vi "SEWV Specific Enthalpy of Water Vapor Revised (J to Kg).vi"(2 "Partial Pressure of Water Vapor":dbl[unit], 3 "Tceg":dbl[unit]) -> (0 "Spesific Valume":dbl[unit], 1 "SEWV":dbl[unit])   [LabVIEW 2018]
panel:
  out "Spesific Vaolume":dbl[unit](slide) scale=0.0..100.0
  out "SEWV":dbl[unit](knob) scale=0.0..6000000.0
  out "DriveGamaRTconstant":dbl
  out "DriveGama0Tconstant":dbl
  out "DriveGamaRPconstant":dbl
  out "Partial Presure of Water Vapor":dbl[unit](knob) scale=0.0..2.0
  out "Temprature of Humid Air\nKelvin Degree":dbl[unit](slide) scale=273.0..373.0
  out "Tk":dbl[unit]
  out "DriveGama0Pconstant":dbl
  out "Temprature of Humid Air\nCentigrade Degree":dbl[unit](slide) scale=0.0..100.0
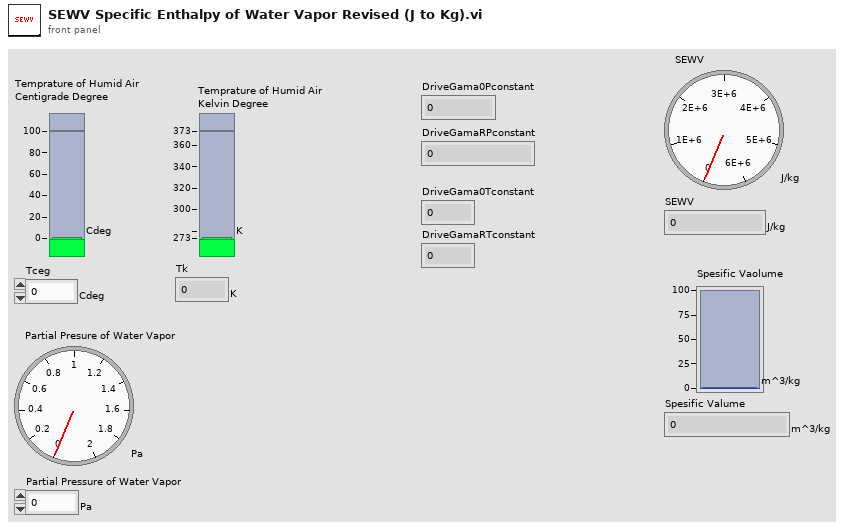
[diagram p1: front panel]
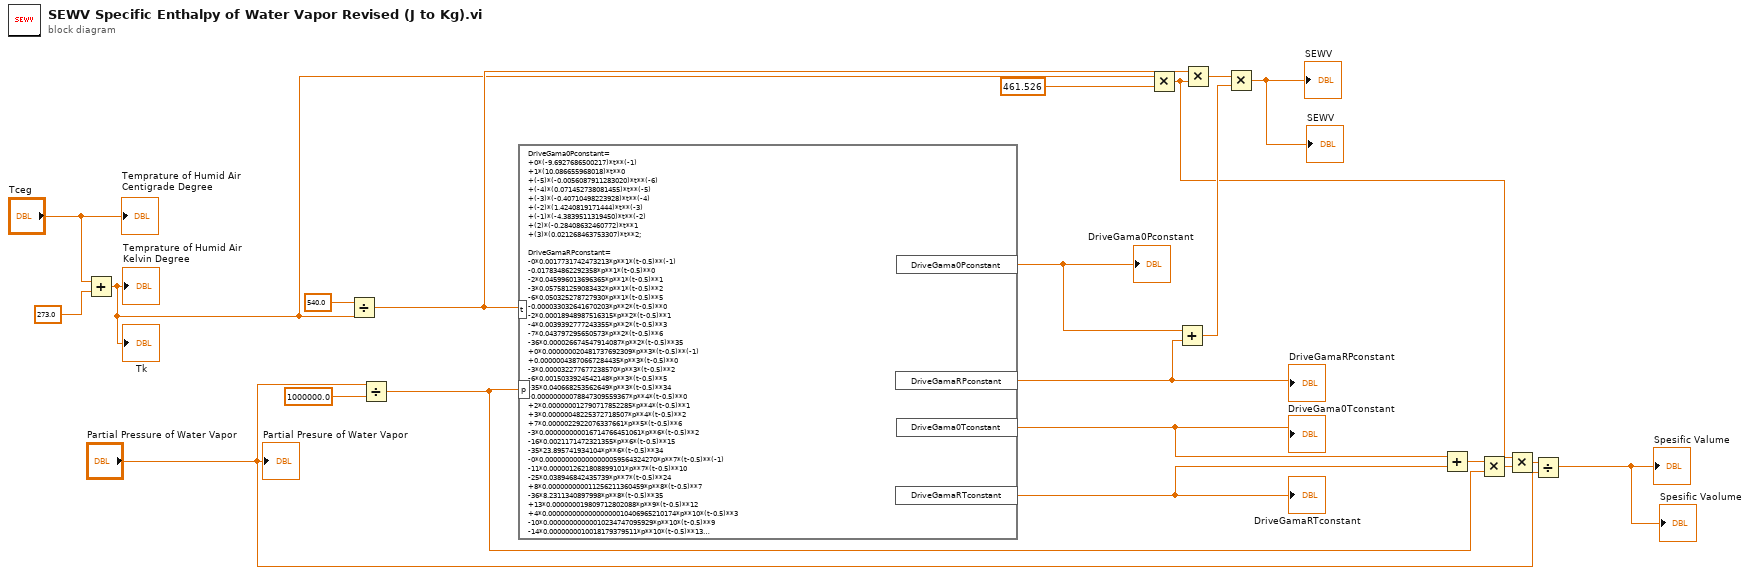
[diagram p0: block diagram]
diagram:
  n1 = Add(x="Tceg", y=dbl[unit] 273.0) -> (x+y=w6:dbl[unit])
  "Tk" <- w6
  "Temprature of Humid Air\nKelvin Degree" <- w6
  n2 = Divide(x=dbl[unit] 540.0, y=w6) -> (x/y=w12:dbl)
  n3 = Divide(x="Partial Pressure of Water Vapor", y=dbl[unit] 1000000.0) -> (x/y=w8:dbl)
  n4 = formula code="DriveGama0Pconstant=\n+0*(-9.6927686500217)*t**(-1)\n+1*(10.086655968018)*t**0\n+(-5)*(-0.0056087911283020)*t**(-6)\n+(-4)*(0.071452738081455)*t**(-5)\n+(-3)*(-0.40710498223928)*t**(-4)\n+(-2)*(1.4240819171444)*t**(-3)\n+(-1)*(-4.3839511319450)*t**(-2)\n+(2)*(-0.28408632460772)*t**1\n+(3)*(0.021268463753307)*t**2;\n\nDriveGamaRPconstant=\n-0*0.0017731742473213*p**1*(t-0.5)**(-1)\n-0.017834862292358*p**1*(t-0.5)**0\n-2*0.045996013696365*p**1*(t-0.5)**1\n-3*0.057581259083432*p**1*(t-0.5)**2\n-6*0.050325278727930*p**1*(t-0.5)**5\n-0.000033032641670203*p**2*(t-0.5)**0\n-2*0.00018948987516315*p**2*(t-0.5)**1\n-4*0.0039392777243355*p**2*(t-0.5)**3\n-7*0.043797295650573*p**2*(t-0.5)**6\n-36*0.000026674547914087*p**2*(t-0.5)**35\n+0*0.000000020481737692309*p**3*(t-0.5)**(-1)\n+0.00000043870667284435*p**3*(t-0.5)**0\n-3*0.000032277677238570*p**3*(t-0.5)**2\n-6*0.0015033924542148*p**3*(t-0.5)**5\n-35*0.040668253562649*p**3*(t-0.5)**34\n-0.00000000078847309559367*p**4*(t-0.5)**0\n+2*0.000000012790717852285*p**4*(t-0.5)**1\n+3*0.00000048225372718507*p**4*(t-0.5)**2\n+7*0.0000022922076337661*p**5*(t-0.5)**6\n-3*0.000000000016714766451061*p**6*(t-0.5)**2\n-16*0.0021171472321355*p**6*(t-0.5)**15\n-35*23.895741934104*p**6*(t-0.5)**34\n-0*0.0000000000000000059564324270*p**7*(t-0.5)**(-1)\n-11*0.0000012621808899101*p**7*(t-0.5)**10\n-25*0.038946842435739*p**7*(t-0.5)**24\n+8*0.000000000011256211360459*p**8*(t-0.5)**7\n-36*8.2311340897998*p**8*(t-0.5)**35\n+13*0.000000019809712802088*p**9*(t-0.5)**12\n+4*0.00000000000000000010406965210174*p**10*(t-0.5)**3\n-10*0.00000000000010234747095929*p**10*(t-0.5)**9\n-14*0.0000000010018179379511*p**10*(t-0.5)**13\n-29*0.000000000080882908646985*p**16*(t-0.5)**28\n+50*0.10693031879409*p**16*(t-0.5)**49\n-57*0.33662250574171*p**18*(t-0.5)**56\n+20*0.00000000000000000000000089185845355421*p**20*(t-0.5)**19\n+35*0.00000000000030629306876232*p**20*(t-0.5)**34\n-48*0.42002467698208*10**(-5)*p**20*(t-0.5)**47\n-21*0.59056029685639*10**(-25)*p**21*(t-0.5)**20\n+53*0.37826947613457*10**(-5)*p**22*(t-0.5)**52\n-39*0.12768608934681*10**(-14)*p**23*(t-0.5)**38\n+26*0.73087610595061*10**(-28)*p**24*(t-0.5)**25\n+40*0.55414715350778*10**(-16)*p**24*(t-0.5)**39\n-58*0.94369707241210*10**(-6)*p**24*(t-0.5)**57;\n\nDriveGama0Tconstant=1/p;\n\nDriveGamaRTconstant=\n-0.17731742473213*10**(-2)*p**0*(t-0.5)**0\n-0.17834862292358*10**(-1)*p**0*(t-0.5)**1\n-0.45996013696365*10**(-1)*p**0*(t-0.5)**2\n-0.57581259083432*10**(-1)*p**0*(t-0.5)**3\n-0.50325278727930*10**(-1)*p**0*(t-0.5)**6\n-2*0.33032641670203*10**(-4)*p**1*(t-0.5)**1\n-2*0.18948987516315*10**(-3)*p**1*(t-0.5)**2\n-2*0.39392777243355*10**(-2)*p**1*(t-0.5)**4\n-2*0.43797295650573*10**(-1)*p**1*(t-0.5)**7\n-2*0.26674547914087*10**(-4)*p**1*(t-0.5)**36\n+3*0.20481737692309*10**(-7)*p**2*(t-0.5)**0\n+3*0.43870667284435*10**(-6)*p**2*(t-0.5)**1\n-3*0.32277677238570*10**(-4)*p**2*(t-0.5)**3\n-3*0.15033924542148*10**(-2)*p**2*(t-0.5)**6\n-3*0.40668253562649*10**(-1)*p**2*(t-0.5)**35\n-4*0.78847309559367*10**(-9)*p**3*(t-0.5)**1\n+4*0.12790717852285*10**(-7)*p**3*(t-0.5)**2\n+4*0.48225372718507*10**(-6)*p**3*(t-0.5)**3\n+5*0.22922076337661*10**(-5)*p**4*(t-0.5)**7\n-6*0.16714766451061*10**(-10)*p**5*(t-0.5)**3\n-6*0.21171472321355*10**(-2)*p**5*(t-0.5)**16\n-6*0.23895741934104*10**(2)*p**5*(t-0.5)**35\n-7*0.59059564324270*10**(-17)*p**6*(t-0.5)**0\n-7*0.12621808899101*10**(-5)*p**6*(t-0.5)**11\n-7*0.38946842435739*10**(-1)*p**6*(t-0.5)**25\n+8*0.11256211360459*10**(-10)*p**7*(t-0.5)**8\n-8*0.82311340897998*10**(1)*p**7*(t-0.5)**36\n+9*0.19809712802088*10**(-7)*p**8*(t-0.5)**13\n+10*0.10406965210174*10**(-18)*p**9*(t-0.5)**4\n-10*0.10234747095929*10**(-12)*p**9*(t-0.5)**10\n-10*0.10018179379511*10**(-8)*p**9*(t-0.5)**14\n-16*0.80882908646985*10**(-10)*p**15*(t-0.5)**29\n+16*0.10693031879409*10**(0)*p**15*(t-0.5)**50\n-18*0.33662250574171*10**(0)*p**17*(t-0.5)**57\n+20*0.89185845355421*10**(-24)*p**19*(t-0.5)**20\n+20*0.30629306876232*10**(-12)*p**19*(t-0.5)**35\n-20*0.42002467698208*10**(-5)*p**19*(t-0.5)**48\n-21*0.59056029685639*10**(-25)*p**20*(t-0.5)**21\n+22*0.37826947613457*10**(-5)*p**21*(t-0.5)**53\n-23*0.12768608934681*10**(-14)*p**22*(t-0.5)**39\n+24*0.73087610595061*10**(-28)*p**23*(t-0.5)**26\n+24*0.55414715350778*10**(-16)*p**23*(t-0.5)**40\n-24*0.94369707241210*10**(-6)*p**23*(t-0.5)**58;"("t"=w12, "p"=w8) -> ("DriveGama0Pconstant"=w17:dbl, "DriveGamaRPconstant"=w16:dbl, "DriveGama0Tconstant"=w11:dbl, "DriveGamaRTconstant"=w10:dbl)
  "DriveGama0Pconstant" <- w17
  "DriveGamaRPconstant" <- w16
  "DriveGama0Tconstant" <- w11
  "DriveGamaRTconstant" <- w10
  n5 = Multiply(x=w6, y=dbl[unit] 461.526) -> (x*y=w3:dbl[unit])
  n6 = Add(x=w17, y=w16) -> (x+y=w13:dbl)
  n7 = Multiply(x=w12, y=w3) -> (x*y=w14:dbl[unit])
  n8 = Multiply(x=w14, y=w13) -> (x*y=→"SEWV" →"SEWV":dbl[unit])
  n9 = Add(x=w11, y=w10) -> (x+y=w9:dbl)
  n10 = Multiply(x=w9, y=w8) -> (x*y=w7:dbl)
  n11 = Multiply(x=w3, y=w7) -> (x*y=w5:dbl[unit])
  n12 = Divide(x=w5, y="Partial Pressure of Water Vapor") -> (x/y=→"Spesific Valume" →"Spesific Vaolume":dbl[unit])
  "Temprature of Humid Air\nCentigrade Degree" <- "Tceg"
  "Partial Presure of Water Vapor" <- "Partial Pressure of Water Vapor"
